vi "Broad Humidity. Data.vi"(8 "error in":errorcluster, 10 "Humidity Data":T1) -> (0 "error out":errorcluster)   [LabVIEW 2021, in "Environment Chamber.lvlib"]
doc: "_____\nCreated using DQMH Event Scripter 6.1.0.128."
uses:
  Environment Chamber.lvlib
  Broad Humidity. Data Argument--cluster.ctl
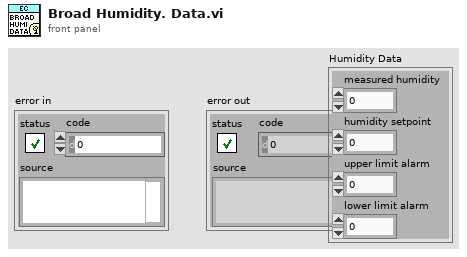
[diagram p1: front panel]
types:
  T1 = cluster{"measured humidity":dbl, "humidity setpoint":dbl, "upper limit alarm":dbl, "lower limit alarm":dbl}
  T2 = typedef "Environment Chamber.lvlib/Broad Humidity. Data Argument--cluster.ctl" = cluster{"Boolean":bool, "Humidity Data":cluster{"measured humidity":dbl, "humidity setpoint":dbl, "upper limit alarm":dbl, "lower limit alarm":dbl}}
  T3 = typedef "Environment Chamber.lvlib/Broadcast Events--cluster.ctl" = cluster{"Module Did Init":refnum<user-event>, "Status Updated":refnum<user-event>, "Error Reported":refnum<user-event>, "Module Did Stop":refnum<user-event>, "Update Module Execution Status":refnum<user-event>, "Broad Temp Data":refnum<user-event>, "Broad Humidity. Data":refnum<user-event>}
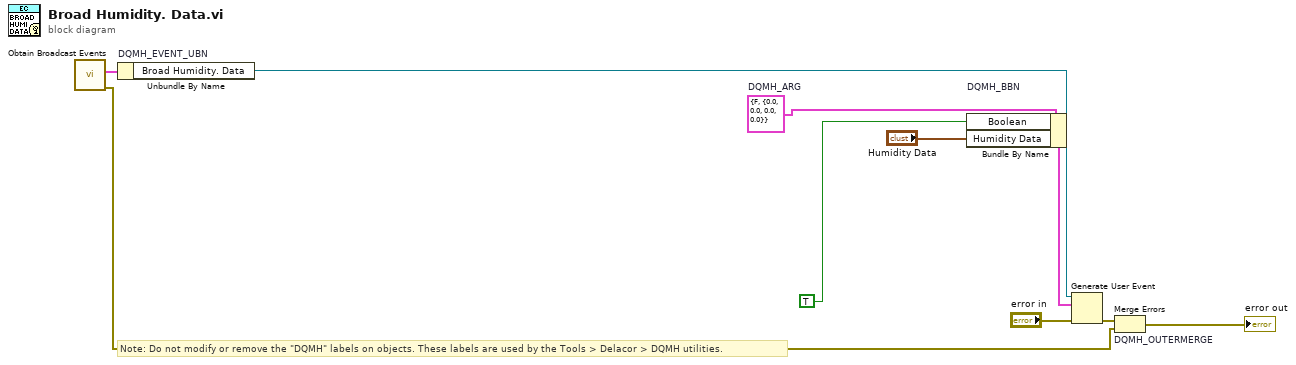
[diagram p0: block diagram]
diagram:
  w5 = T2 {"Boolean"=FALSE, "Humidity Data"={"measured humidity"=0.0, "humidity setpoint"=0.0, "upper limit alarm"=0.0, "lower limit alarm"=0.0}}  # DQMH_ARG
  # "Note: Do not modify or remove the \"DQMH\" labels on objects. These labels are used by the Tools > Delacor > DQMH utilities."
  n1 = call "Obtain Broadcast Events.vi"() -> ("error out"=w3:errorcluster, "Environment Chamber Broadcast Events"=w2:T3)  [unwired: 10 in]
  n2 = Unbundle By Name "DQMH_EVENT_UBN"(w2) -> ("Broad Humidity. Data"=w7:refnum<user-event>)
  n3 = Bundle By Name "DQMH_BBN"(cluster=w5, "Boolean"=TRUE, "Humidity Data"="Humidity Data") -> (w8:T2)
  n4 = Generate User Event(user event=w7, event data cluster=w8, error in="error in") -> (error out=w6:errorcluster)  [unwired: 1 in, 1 out]
  n5 = Merge Errors "DQMH_OUTERMERGE"(w6, w3) -> (→"error out":errorcluster)
